vi "EEI EXP11.vi"() -> ()   [LabVIEW 2020]
panel:
  out "output array":dbl[](array[numeric])
  in  "Numeric":i32
  out "Waveform Graph":dbl[](graph)
  out "Waveform Chart":dbl[](graph)
  in  "Frequency":dbl
  in  "Amplitude":dbl
  in  "Time":i32
  out "current time":timestamp
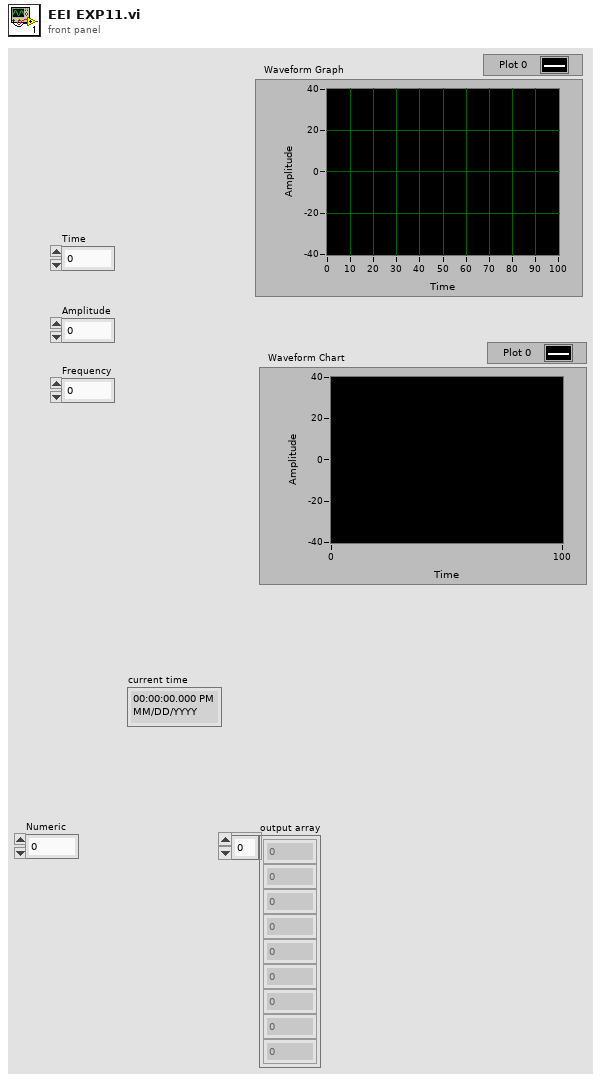
[diagram p1: front panel]
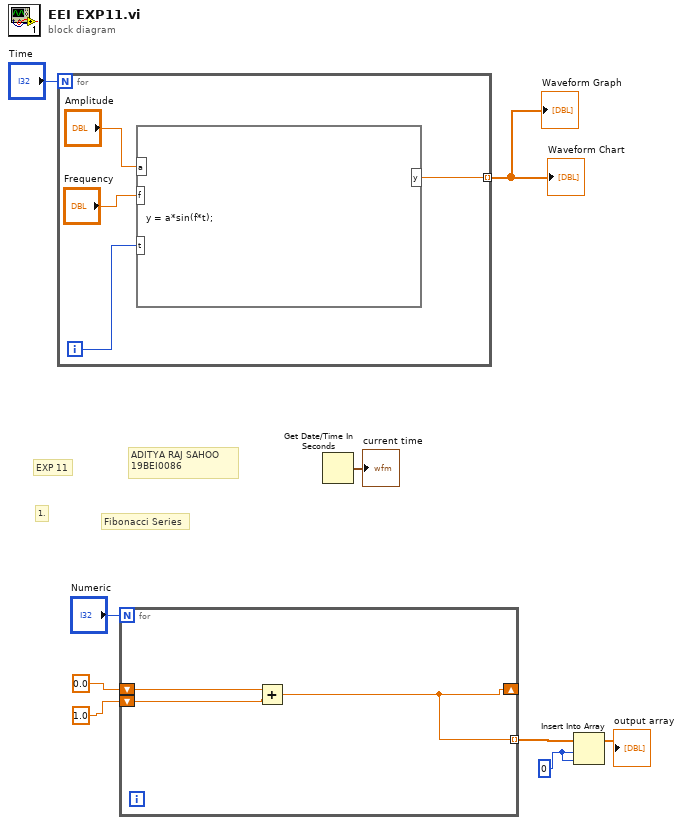
[diagram p0: block diagram]
diagram:
  w4 = 0 ("index")
  # "Fibonacci Series"
  # "1."
  # "ADITYA RAJ SAHOO\n19BEI0086"
  # "EXP 11"
  n1 = for {
    N: "Time" -> [_]
    tunnel: [w10] -> w7 mode=indexing
    i -> [w11]
    n2 = formula code="y = a*sin(f*t);"("a"="Amplitude", "f"="Frequency", "t"=w11) -> ("y"=w10:dbl)
  }
  "Waveform Chart" <- w7
  "Waveform Graph" <- w7
  n3 = for {
    N: "Numeric" -> [_]
    shift-right: [w15] -> _
    shift-left: 0.0 ("x") -> [w16]
    tunnel: [w15] -> w3 mode=indexing
    shift-left: 1.0 ("y") -> [w14]
    n4 = Add(x=w16, y=w14) -> (x+y=w15:dbl)
  }
  n5 = Get Date/Time In Seconds() -> (seconds since 1Jan1904=→"current time":timestamp)
  n6 = Insert Into Array(array=w3, index=w4, new element=w4) -> (→"output array":dbl[])
